vi "Configure Window Timebase.vi"(8 "error in (no error)":errorcluster, 9 "Range (5.0E-6)":dbl=5e-06, 10 "Position (0.0 s)":dbl, 11 "VISA resource name":refnum<visa-resource-name>) -> (0 "error out":errorcluster, 3 "VISA resource name out":refnum<visa-resource-name>)   [LabVIEW 2017, in "Agilent 6000 Series.lvlib"]
doc: "This VI configures the properties that control the time base window. These properties are the time base position and range.\n\n<B>Note:</B>\n\n(1) This VI has been obsoleted from the driver and is included for compatibility with existing applications. New applications should use the <B>Configure Timebase Mode</B> VI."
uses:
  <instrlib>/Agilent 6000 Series/Agilent 6000 Series.lvlib
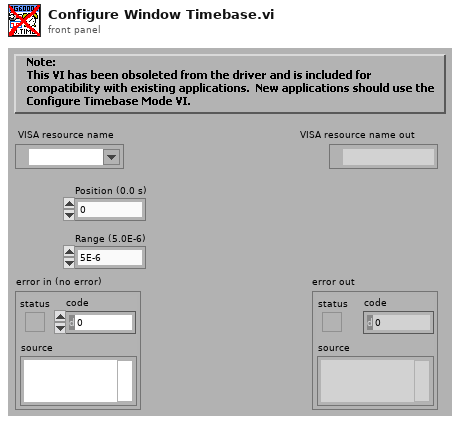
[diagram p1: front panel]
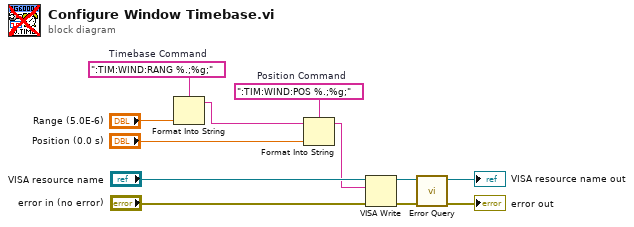
[diagram p0: block diagram]
diagram:
  w5 = ":TIM:WIND:POS %.;%g;"  # Position Command
  w6 = ":TIM:WIND:RANG %.;%g;"  # Timebase Command
  n1 = Format Into String(format string=w6, "Range (5.0E-6)") -> (resulting string=w4:string)  [unwired: 2 in, 1 out]
  n2 = Format Into String(format string=w5, initial string=w4, "Position (0.0 s)") -> (resulting string=w2:string)  [unwired: 1 in, 1 out]
  n3 = VISA Write(VISA resource name="VISA resource name", write buffer=w2, error in (no error)="error in (no error)") -> (VISA resource name out=w8:refnum<visa-resource-name>, error out=w7:errorcluster)  [unwired: 1 out]
  n4 = call <instrlib>:"Error Query.vi"("error in (no error)"=w7, "VISA resource name"=w8) -> ("error out"=→"error out":errorcluster, "VISA resource name out"=→"VISA resource name out":refnum<visa-resource-name>)  [unwired: 6 in, 2 out]
